vi "Test Initialise.vi"(11 "Test Case In":refnum<class "Sprite Font Tests.lvclass">) -> (0 "error out":errorcluster, 3 "Test Case Out":refnum<class "Sprite Font Tests.lvclass">)   [LabVIEW 2021, in "Sprite Font Tests.lvclass"]
uses:
  Sprite Font Tests.lvclass
  Sprite Font Tests.lvclass/Sprite Font Tests.ctl
  Application Specific/Renderer/Renderer.lvclass
  <vilib>/Astemes/LUnit/Test Case.lvclass
  Application Specific/Sprite Font/Sprite Font.lvclass
  Application Specific/Resource Manager/Resource Manager.lvclass
  Application Specific/Sprite Font/Game Font.ctl
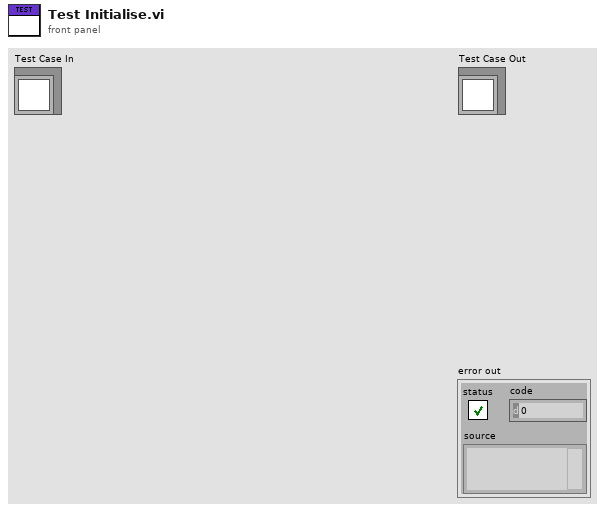
[diagram p1: front panel]
types:
  T1 = typedef "Sprite Font.lvclass/Game Font.ctl" = enum16{"Ilwrath", "Micro", "Slylandro", "Starcon", "Tiny", "Utwig"}
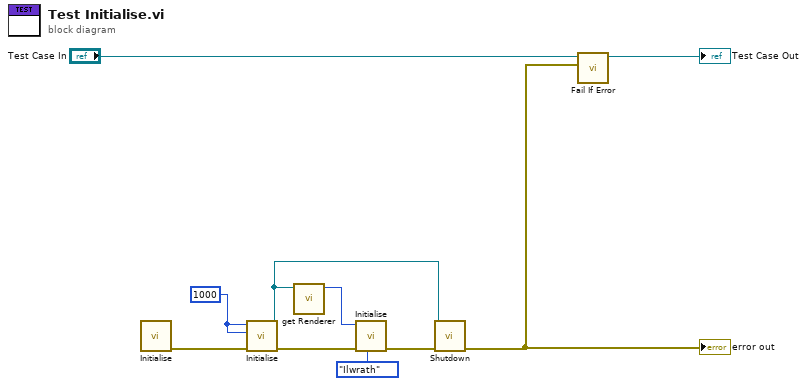
[diagram p0: block diagram]
diagram:
  w7 = 1000 ("Width")
  n1 = call "Initialise.vi"() -> ("error out"=w2:errorcluster)  [unwired: 11 in]
  n2 = call "Initialise.vi"("error in (no error)"=w2, "Window Height"=w7, "Window Width"=w7) -> ("error out"=w6:errorcluster, "Renderer out"=w4:refnum<class "Renderer.lvclass">)  [unwired: 7 in]
  n3 = call-dynamic "get Renderer.vi"("Renderer in"=w4) -> ("Renderer"=w3:u32)  [unwired: 10 in]
  n4 = call "Initialise.vi"("Font"=Game_Font."Ilwrath", "error in (no error)"=w6, "Renderer"=w3) -> ("error out"=w5:errorcluster)  [unwired: 7 in, 1 out]
  n5 = call "Shutdown.vi"("error in (no error)"=w5, "Renderer"=w4) -> ("error out"=w8:errorcluster)  [unwired: 9 in]
  "error out" <- w8
  n6 = call <vilib>:"Fail If Error.vi"("Assert error"=w8, "LUnit Test Case In"="Test Case In") -> ("LUnit Test Case Out"=→"Test Case Out":refnum<class "Sprite Font Tests.lvclass">)  [unwired: 8 in, 1 out]
